vi "GET_Running_perc._travel_and_avg._speed_(online).vi"(8 "Reset? (F)":bool, 9 "Animal coordinates in":T1, 10 "Histogram parameters":T3, 11 "Running stats results in":T2) -> (3 "Running stats results out":T2)   [LabVIEW 2018, in "Tracker.lvlib"]
uses:
  Tracker.lvlib
  Controls/CTL_Histogram_parameters.ctl
  Controls/CTL_Running_statistics_results.ctl
  Controls/CTL_Animal_Coordinates_and_Speed.ctl
  Common_Resources.lvlib
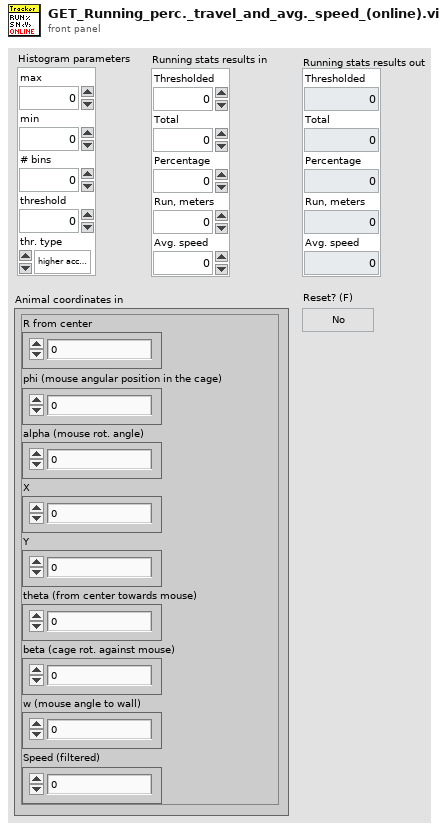
[diagram p1: front panel]
types:
  T1 = typedef "Common_Resources.lvlib/CTL_Animal_Coordinates_and_Speed.ctl" = cluster{"R from center":dbl, "phi (mouse angular position in the cage)":dbl, "alpha (mouse rot. angle)":dbl, "X":dbl, "Y":dbl, "theta (from center towards mouse)":dbl, "beta (cage rot. against mouse)":dbl, "w (mouse angle to wall)":dbl, "Speed (filtered)":dbl}
  T2 = typedef "Common_Resources.lvlib/CTL_Running_statistics_results.ctl" = cluster{"Thresholded":u32, "Total":u32, "Percentage":dbl, "Run, meters":dbl, "Avg. speed":dbl}
  T3 = typedef "Common_Resources.lvlib/CTL_Histogram_parameters.ctl" = cluster{"max":dbl, "min":dbl, "# bins":i32, "threshold":dbl, "thr. type":enum16{"higher accepted", "lower accepted"}}
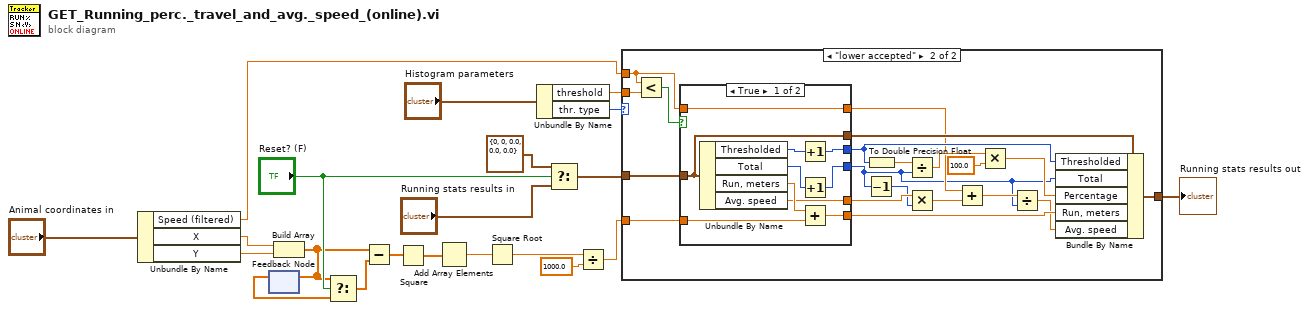
[diagram p0: block diagram]
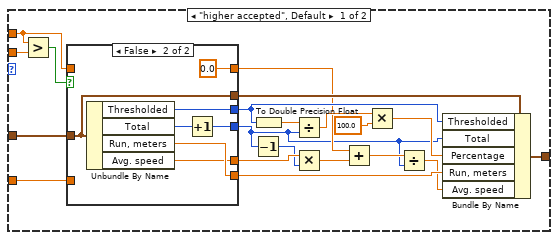
[diagram p2: hidden frame]
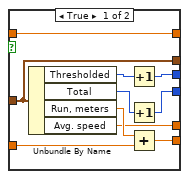
[diagram p3: hidden frame]
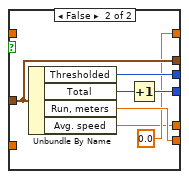
[diagram p4: hidden frame]
diagram:
  n1 = Unbundle By Name("Animal coordinates in") -> ("Speed (filtered)"=w15:dbl, "X"=w14:dbl, "Y"=w13:dbl)
  n2 = feedback #1() -> (w12:dbl[])  [unwired: 1 in]
  n3 = Build Array(w14, w13) -> (w6:dbl[])
  n4 = feedback-in #1(w6) -> ()
  n5 = Select(t=w6, s="Reset? (F)", f=w12) -> (s? t:f=w8:dbl[])
  n6 = Subtract(x=w6, y=w8) -> (x-y=w11:dbl[])
  n7 = Square(x=w11) -> (x^2=w10:dbl[])
  n8 = Add Array Elements(numeric array=w10) -> (sum=w9:dbl)
  n9 = Square Root(x=w9) -> (sqrt(x)=w4:dbl)
  n10 = Unbundle By Name("Histogram parameters") -> ("threshold"=w19:dbl, "thr. type"=w20:enum16{"higher accepted", "lower accepted"})
  n11 = Select(t=T2 {"Thresholded"=0, "Total"=0, "Percentage"=0.0, "Run, meters"=0.0, "Avg. speed"=0.0} ("Running stats results"), s="Reset? (F)", f="Running stats results in") -> (s? t:f=w18:T2)
  n12 = Divide(x=w4, y=1000.0) -> (x/y=w1:dbl)
  n13 = case shown="\"lower accepted\"" w20 {
    tunnel: w15 -> [w29 w66]
    tunnel: w19 -> [w41 w78]
    tunnel: w18 -> [w32 w69]
    tunnel: [w33 w70] -> w2
    tunnel: w1 -> [w30 w67]
    frame "higher accepted", Default {
      n14 = Greater?(x=w29, y=w41) -> (0:w40:bool)
      n15 = case shown="False" w40 {
        tunnel: w32 -> [w47 w55]
        tunnel: [w49 w57] -> w23
        tunnel: [w48 w56] -> w34
        tunnel: [w47 w55] -> w36
        tunnel: [w44 w54] -> w31
        tunnel: w30 -> [w46 _]
        tunnel: w29 -> [w43 _]
        tunnel: [w43 0.0 ("Speed (filtered)")] -> w28
        tunnel: [w42 w52] -> w26
        frame True {
          n16 = Unbundle By Name(w47) -> ("Thresholded"=w51:u32, "Total"=w50:u32, "Run, meters"=w45:dbl, "Avg. speed"=w42:dbl)
          n17 = Increment(x=w51) -> (x+1=w48:u32)
          n18 = Increment(x=w50) -> (x+1=w49:u32)
          n19 = Add(x=w45, y=w46) -> (x+y=w44:dbl)
        }
        frame False {
          n20 = Unbundle By Name(w55) -> ("Thresholded"=w56:u32, "Total"=w58:u32, "Run, meters"=w54:dbl, "Avg. speed"=w52:dbl)
          n21 = Increment(x=w58) -> (x+1=w57:u32)
        }
      }
      n22 = Decrement(x=w23) -> (x-1=w25:u32)
      n23 = To Double Precision Float(number=w34) -> (double precision float=w39:dbl)
      n24 = Divide(x=w39, y=w23) -> (x/y=w38:dbl)
      n25 = Multiply(x=w26, y=w25) -> (x*y=w27:dbl)
      n26 = Add(x=w28, y=w27) -> (x+y=w24:dbl)
      n27 = Multiply(x=w38, y=100.0) -> (x*y=w35:dbl)
      n28 = Divide(x=w24, y=w23) -> (x/y=w22:dbl)
      n29 = Bundle By Name(cluster=w36, "Thresholded"=w34, "Total"=w23, "Percentage"=w35, "Run, meters"=w31, "Avg. speed"=w22) -> (w33:T2)
    }
    frame "lower accepted" {
      n30 = Less?(x=w66, y=w78) -> (x < y?=w77:bool)
      n31 = case shown="True" w77 {
        tunnel: w69 -> [w84 w92]
        tunnel: [w86 w94] -> w60
        tunnel: [w85 w93] -> w71
        tunnel: [w84 w92] -> w73
        tunnel: [w81 w91] -> w68
        tunnel: w67 -> [w83 _]
        tunnel: w66 -> [w80 _]
        tunnel: [w80 0.0 ("Speed (filtered)")] -> w65
        tunnel: [w79 w89] -> w63
        frame True {
          n32 = Unbundle By Name(w84) -> ("Thresholded"=w88:u32, "Total"=w87:u32, "Run, meters"=w82:dbl, "Avg. speed"=w79:dbl)
          n33 = Increment(x=w88) -> (x+1=w85:u32)
          n34 = Increment(x=w87) -> (x+1=w86:u32)
          n35 = Add(x=w82, y=w83) -> (x+y=w81:dbl)
        }
        frame False {
          n36 = Unbundle By Name(w92) -> ("Thresholded"=w93:u32, "Total"=w95:u32, "Run, meters"=w91:dbl, "Avg. speed"=w89:dbl)
          n37 = Increment(x=w95) -> (x+1=w94:u32)
        }
      }
      n38 = Decrement(x=w60) -> (x-1=w62:u32)
      n39 = To Double Precision Float(number=w71) -> (double precision float=w76:dbl)
      n40 = Divide(x=w76, y=w60) -> (x/y=w75:dbl)
      n41 = Multiply(x=w63, y=w62) -> (x*y=w64:dbl)
      n42 = Add(x=w65, y=w64) -> (x+y=w61:dbl)
      n43 = Multiply(x=w75, y=100.0) -> (x*y=w72:dbl)
      n44 = Divide(x=w61, y=w60) -> (x/y=w59:dbl)
      n45 = Bundle By Name(cluster=w73, "Thresholded"=w71, "Total"=w60, "Percentage"=w72, "Run, meters"=w68, "Avg. speed"=w59) -> (w70:T2)
    }
  }
  "Running stats results out" <- w2
